vi "CH_LM App DataFileRow.vi"(1 "Data format":u16, 2 "Probe Info":cluster{"Probe Type":T2, "Probe Qualifier":T3}[](array[cluster]), 3 "Data Array":T1[](array[typedef]) {"Flags" format="%.0b"; "Unit ID" format="%.0b"; "Quad Distance"."Y" format="%#.1f"; "Quad Distance"."X" format="%#.1f"; "Value" format="%#.7e"}, 4 "Counts String":string) -> (0 "Data Row String":string)   [LabVIEW 2012, in "CH_LM App.lvlib"]
doc: "This VI concenates data to a data row string to be written to file."
uses:
  CH_LM App.lvlib
  CH_LM/CH_LM ProbeType.ctl
  CH_LM.lvlib
  CH_LM/CH_LM ProbeQualifier.ctl
  CH_LM/CH_LM Streaming Data.ctl
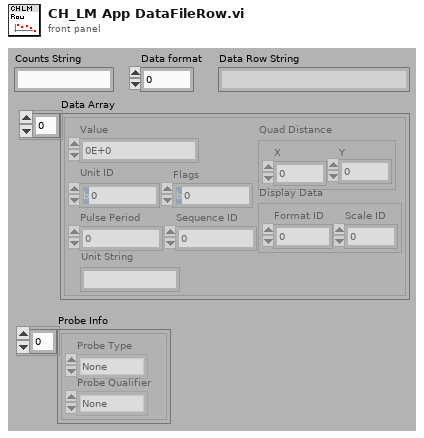
[diagram p1: front panel]
types:
  T1 = typedef "CH_LM.lvlib/CH_LM Streaming Data.ctl" = cluster{"Value":sgl, "Quad Distance":cluster{"X":sgl, "Y":sgl}, "Display Data":cluster{"Format ID":u8, "Scale ID":u8}, "Unit ID":u8, "Flags":u32, "Pulse Period":u32, "Sequence ID":u32, "Unit String":string}
  T2 = typedef "CH_LM.lvlib/CH_LM ProbeType.ctl" = enum16{"None", "Thermopile", "Pyroelectric", "Optical"}
  T3 = typedef "CH_LM.lvlib/CH_LM ProbeQualifier.ctl" = enum16{"None", "Single", "Quad", "No Spec"}
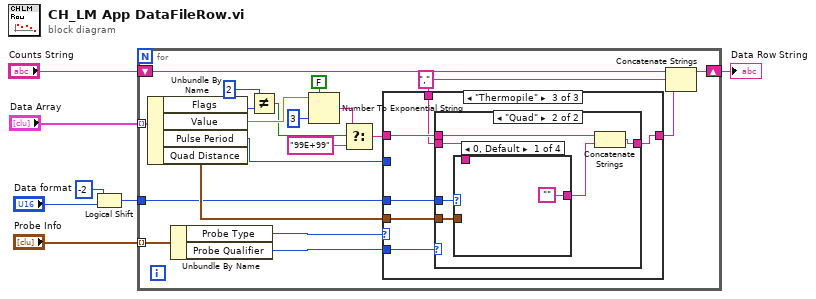
[diagram p0: block diagram]
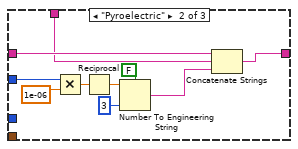
[diagram p3: hidden frame]
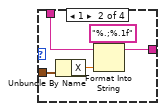
[diagram p5: hidden frame]
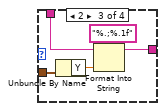
[diagram p6: hidden frame]
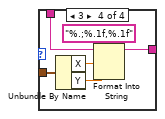
[diagram p7: hidden frame]
diagram:
  n1 = Logical Shift(y=i16 -2, x="Data format") -> (x << y=w2:u16)
  n2 = for {
    shift-right: [w20] -> w6
    shift-left: "Counts String" -> [w22]
    tunnel: "Data Array" -> [w19] mode=indexing
    tunnel: "Probe Info" -> [w18] mode=indexing
    tunnel: w2 -> [w10]
    w17 = "," ("string")
    n3 = Unbundle By Name(w19) -> ("Flags"=w14:u32, "Value"=w27:sgl, "Pulse Period"=w9:u32, "Quad Distance"=w11:cluster{"X":sgl, "Y":sgl})
    n4 = Unbundle By Name(w18) -> ("Probe Type"=w16:T2, "Probe Qualifier"=w12:T3)
    n5 = Not Equal?(x=u8 2 ("Flags"), y=w14) -> (x != y?=w13:bool)
    n6 = Number To Exponential String(number=w27, precision (6)=i16 3, 1:FALSE ("use system decimal point (T)")) -> (E-format string=w25:string)  [unwired: 1 out]
    n7 = Select(t=w25, s=w13, f="99E+99") -> (s? t:f=w8:string)
    n8 = case shown="\"Thermopile\"" w16 {
      tunnel: w8 -> [w28 w38 w44]
      tunnel: [w28 w37 w43] -> w21
      tunnel: w17 -> [_ w36 w42]
      tunnel: w12 -> [_ _ w41]
      tunnel: w11 -> [_ _ w40]
      tunnel: w10 -> [_ _ w39]
      tunnel: w9 -> [_ w32 _]
      frame Default {
      }
      frame "Pyroelectric" {
        n9 = Multiply(x=w32, y=1e-06) -> (x*y=w31:dbl)
        n10 = Reciprocal(x=w31) -> (1/x=w35:dbl)
        n11 = Number To Engineering String(1:FALSE ("use system decimal point (T)"), 2:i16 3 ("precision (6)"), 4:w35) -> (0:w34:string)  [unwired: 1 out]
        n12 = Concatenate Strings(w38, w36, w34) -> (w37:string)
      }
      frame "Thermopile" {
        n13 = case shown="\"Quad\"" w41 {
          tunnel: w44 -> [w45 w51]
          tunnel: [w45 w50] -> w43
          tunnel: w42 -> [_ w46]
          tunnel: w40 -> [_ w49]
          tunnel: w39 -> [_ w47]
          frame "Single", Default {
          }
          frame "Quad" {
            n14 = case shown="0, Default" w47 {
              tunnel: w49 -> [_ w57 w62 w68]
              tunnel: ["" w54 w59 w64] -> w48
              tunnel: w46 -> [_ w53 w58 w63]
              frame 0, Default {
              }
              frame 1 {
                n15 = Unbundle By Name(w57) -> ("X"=w56:sgl)
                n16 = Format Into String(format string="%.;%.1f", initial string=w53, w56) -> (resulting string=w54:string)  [unwired: 1 in, 1 out]
              }
              frame 2 {
                n17 = Unbundle By Name(w62) -> ("Y"=w61:sgl)
                n18 = Format Into String(format string="%.;%.1f", initial string=w58, w61) -> (resulting string=w59:string)  [unwired: 1 in, 1 out]
              }
              frame 3 {
                n19 = Unbundle By Name(w68) -> ("X"=w67:sgl, "Y"=w66:sgl)
                n20 = Format Into String(format string="%.;%.1f,%.1f", initial string=w63, w67, w66) -> (resulting string=w64:string)  [unwired: 1 in, 1 out]
              }
            }
            n21 = Concatenate Strings(w51, w48) -> (w50:string)
          }
        }
      }
    }
    n22 = Concatenate Strings(w22, w17, w21) -> (w20:string)
  }
  "Data Row String" <- w6
